vi "Read Pot Volts.vi"() -> (3 "Encoder Voltages":dbl[](array[numeric]))   [LabVIEW 2020]
uses:
  <vilib>/Rock Robotics/Network Tables/NT Read Boolean.vi
  <vilib>/Rock Robotics/WPI/Utilities/WPI_GetSetVariantRefNum.vi
  <vilib>/Utility/file.llb/Read Delimited Spreadsheet (DBL).vi
  <vilib>/Utility/file.llb/Write Delimited Spreadsheet (DBL).vi
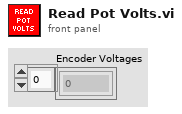
[diagram p1: front panel]
types:
  T1 = typedef "WPI_AnalogChannelDevRef.ctl" = cluster{"DevStatus":errorcluster, "Analog Channel":T2}
  T2 = typedef "FPGA_AIChannel.ctl" = enum8{"AI 0", "AI 1", "AI 2", "AI 3", "AI MXP 0", "AI MXP 1", "AI MXP 2", "AI MXP 3", "Invalid"}
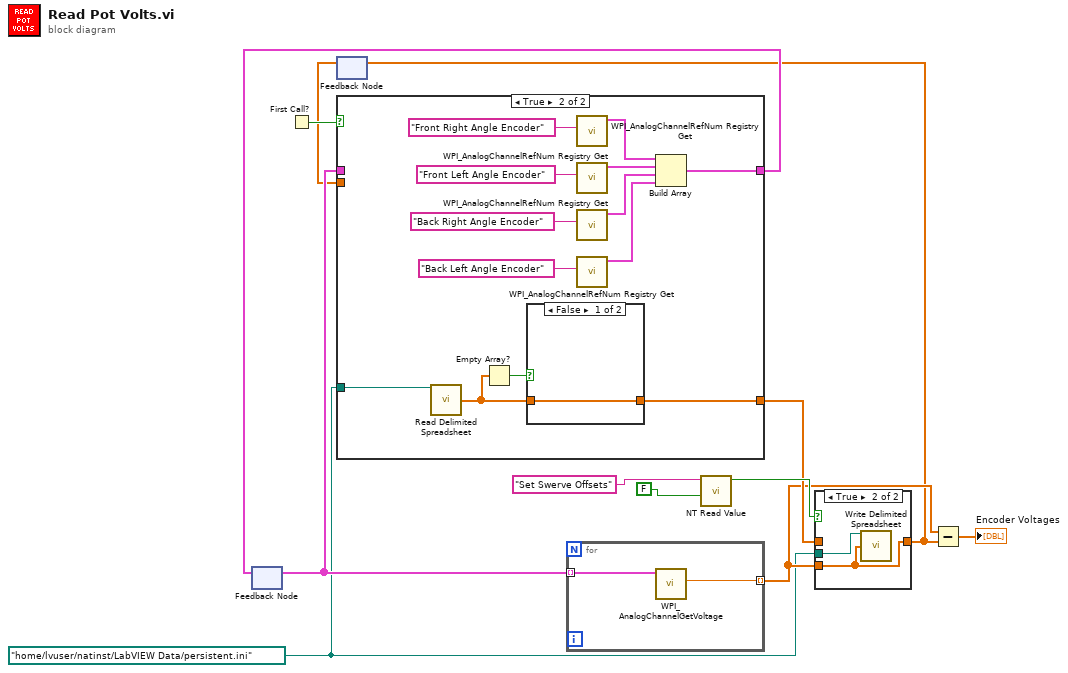
[diagram p0: block diagram]
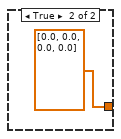
[diagram p4: hidden frame]
diagram:
  w3 = path "/home/lvuser/natinst/LabVIEW Data/persistent.ini" ("file path (dialog if empty)")
  n1 = feedback #1() -> (w10:T1[])  [unwired: 1 in]
  n2 = First Call?() -> (First Call?: T/F=w12:bool)
  n3 = feedback #2() -> (w9:dbl[])  [unwired: 1 in]
  n4 = case shown="True" w12 {
    tunnel: [w14 w27] -> w11
    tunnel: w10 -> [w14 _]
    tunnel: [w13 w21] -> w5
    tunnel: w9 -> [w13 _]
    tunnel: w3 -> [_ w19]
    frame False {
    }
    frame True {
      n5 = call-poly <vilib>:"Read Delimited Spreadsheet.vi"("file path (dialog if empty)"=w19) -> ("first row"=w20:dbl[])  [unwired: 9 in, 5 out]
      n6 = Empty Array?(array=w20) -> (empty?=w22:bool)
      n7 = case shown="False" w22 {
        tunnel: [w28 dbl[] [0.0, 0.0, 0.0, 0.0]] -> w21
        tunnel: w20 -> [w28 _]
        frame False {
        }
        frame True {
        }
      }
      n8 = call <vilib>:"WPI_AnalogChannelRefNum Registry Get.vi"("refnum name"="Front Right Angle Encoder") -> ("AIDeviceRef"=w18:T1)  [unwired: 9 in, 1 out]
      n9 = call <vilib>:"WPI_AnalogChannelRefNum Registry Get.vi"("refnum name"="Front Left Angle Encoder") -> ("AIDeviceRef"=w16:T1)  [unwired: 9 in, 1 out]
      n10 = call <vilib>:"WPI_AnalogChannelRefNum Registry Get.vi"("refnum name"="Back Right Angle Encoder") -> ("AIDeviceRef"=w15:T1)  [unwired: 9 in, 1 out]
      n11 = call <vilib>:"WPI_AnalogChannelRefNum Registry Get.vi"("refnum name"="Back Left Angle Encoder") -> ("AIDeviceRef"=w17:T1)  [unwired: 9 in, 1 out]
      n12 = Build Array(w18, w16, w15, w17) -> (w27:T1[])
    }
  }
  n13 = feedback-in #1(w11) -> ()
  n14 = for {
    tunnel: w10 -> [w30] mode=indexing
    tunnel: [w31] -> w4 mode=indexing
    n15 = call <vilib>:"WPI_AnalogChannelGetVoltage.vi"("AIDeviceRef"=w30) -> ("Voltage"=w31:dbl)  [unwired: 8 in, 2 out]
  }
  n16 = call-poly <vilib>:"NT Read Value.vi"("Default Value"=FALSE, "Name"="Set Swerve Offsets") -> ("Boolean"=w6:bool)  [unwired: 8 in, 1 out]
  n17 = case shown="True" w6 {
    tunnel: [w32 w33] -> w1
    tunnel: w5 -> [w32 _]
    tunnel: w4 -> [_ w33]
    tunnel: w3 -> [_ w34]
    frame False {
    }
    frame True {
      n18 = call-poly <vilib>:"Write Delimited Spreadsheet.vi"("file path (dialog if empty)"=w34, "1D data"=w33) -> ()  [unwired: 12 in, 2 out]
    }
  }
  n19 = feedback-in #2(w1) -> ()
  n20 = Subtract(x=w4, y=w1) -> (x-y=→"Encoder Voltages":dbl[])
